vi "2D_Histogram_Selection.vi"() -> ()   [LabVIEW 2009]
uses:
  <vilib>/Utility/file.llb/Read From Spreadsheet File (DBL).vi
  <vilib>/Utility/file.llb/Write To Spreadsheet File (DBL).vi
panel:
  out "transposed array":dbl[][](array[numeric])
  out "array w/ subset deleted":dbl[](array[numeric])
  out "deleted portion":dbl[](array[numeric])
  in  "1-D Histogram?":bool
  out "1-D Histogram":cluster{dbl[], dbl[]}(graph)
  in  "Result File Dir":path=path "C:/Users/Habid/Documents/08_22_2013/08_22_2013/c6/25.7mV_3RR_2kHz_100mv_MC900/bcurve_selection_0.4"
  in  "Result File Name":string="beta_Histogram.txt"
  in  "Save 1-D":bool
  out "x+1":i32
  out "Cursor.Cursor Index 2":i32
  out "Cursor.Cursor Index":i32
  out "element":dbl
  out "Cursor.Cursor Position:Cursor X":dbl
  in  "Save":bool
  in  "Result File Name 2":string="1D_Histogram.txt"
  in  "Result File Dir 2":path
  out "Result":dbl[][](array[numeric])
  out "Row":i32
  out "Cursor 3":T1 {"Cursor.Cursor Z" format="%.2f"; "Cursor.Cursor Y" format="%.2f"; "Cursor.Cursor X" format="%.2f"}
  out "Cursor 2":T1 {"Cursor.Cursor Z" format="%.2f"; "Cursor.Cursor Y" format="%.2f"; "Cursor.Cursor X" format="%.2f"}
  out "Total 2D Histogram":dbl[][](graph)
  in  "Filename":path=path "C:/Users/Habid/Documents/08_22_2013/08_22_2013/c6/25.7mV_3RR_2kHz_100mv_MC900/bcurve_selection_0.4/2D_Histogram.txt"
  out "Cursor 0":T1 {"Cursor.Cursor Z" format="%.2f"; "Cursor.Cursor Y" format="%.2f"; "Cursor.Cursor X" format="%.2f"}
  out "Cursor 1":T1 {"Cursor.Cursor Z" format="%.2f"; "Cursor.Cursor Y" format="%.2f"; "Cursor.Cursor X" format="%.2f"}
  out "Intensity Graph":dbl[][](graph)
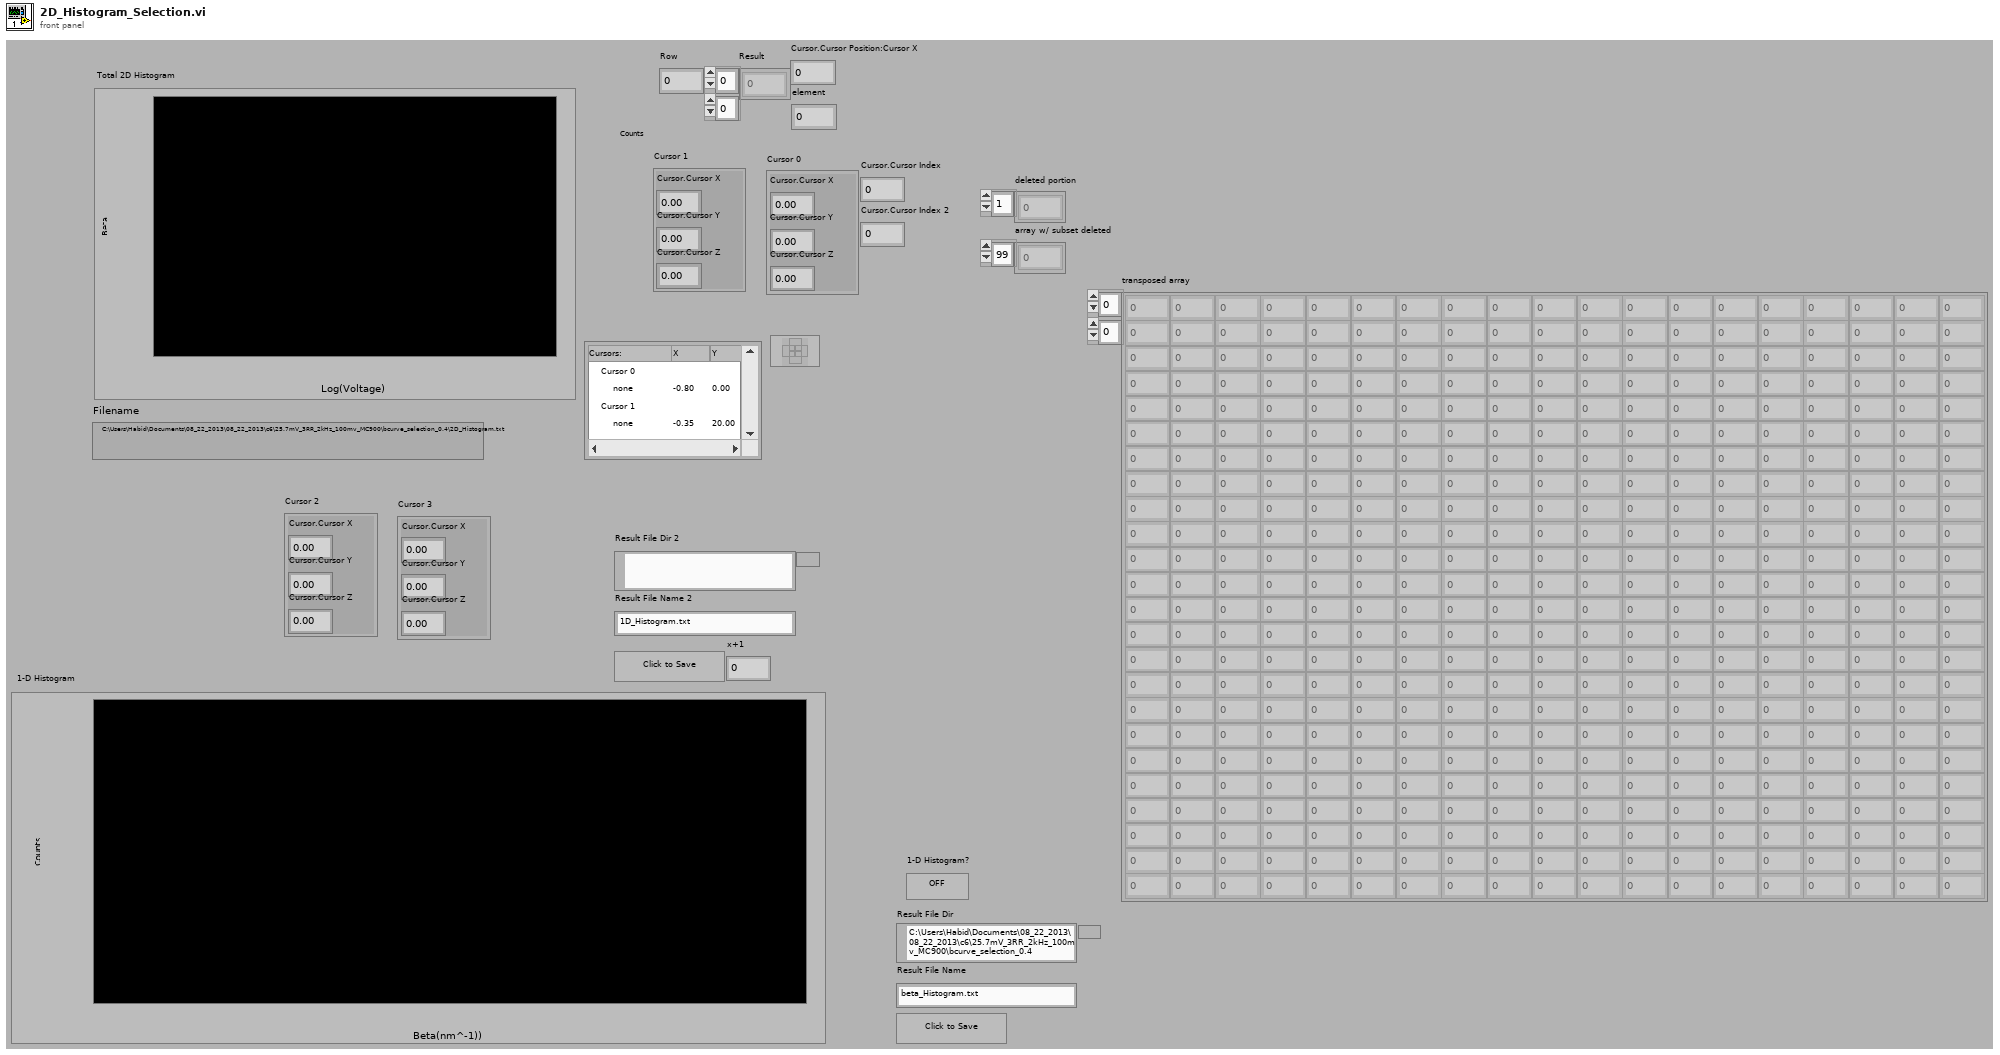
[diagram p1: front panel]
types:
  T1 = cluster{"Cursor.Cursor X":dbl, "Cursor.Cursor Y":dbl, "Cursor.Cursor Z":dbl}
  T2 = cluster{"Cursor.Cursor X":dbl, "Cursor.Cursor Y":dbl, dbl}
  T3 = cluster{"Cursor.Cursor X":dbl, "Cursor.Cursor Y":dbl, "number: 0 to 1":dbl}
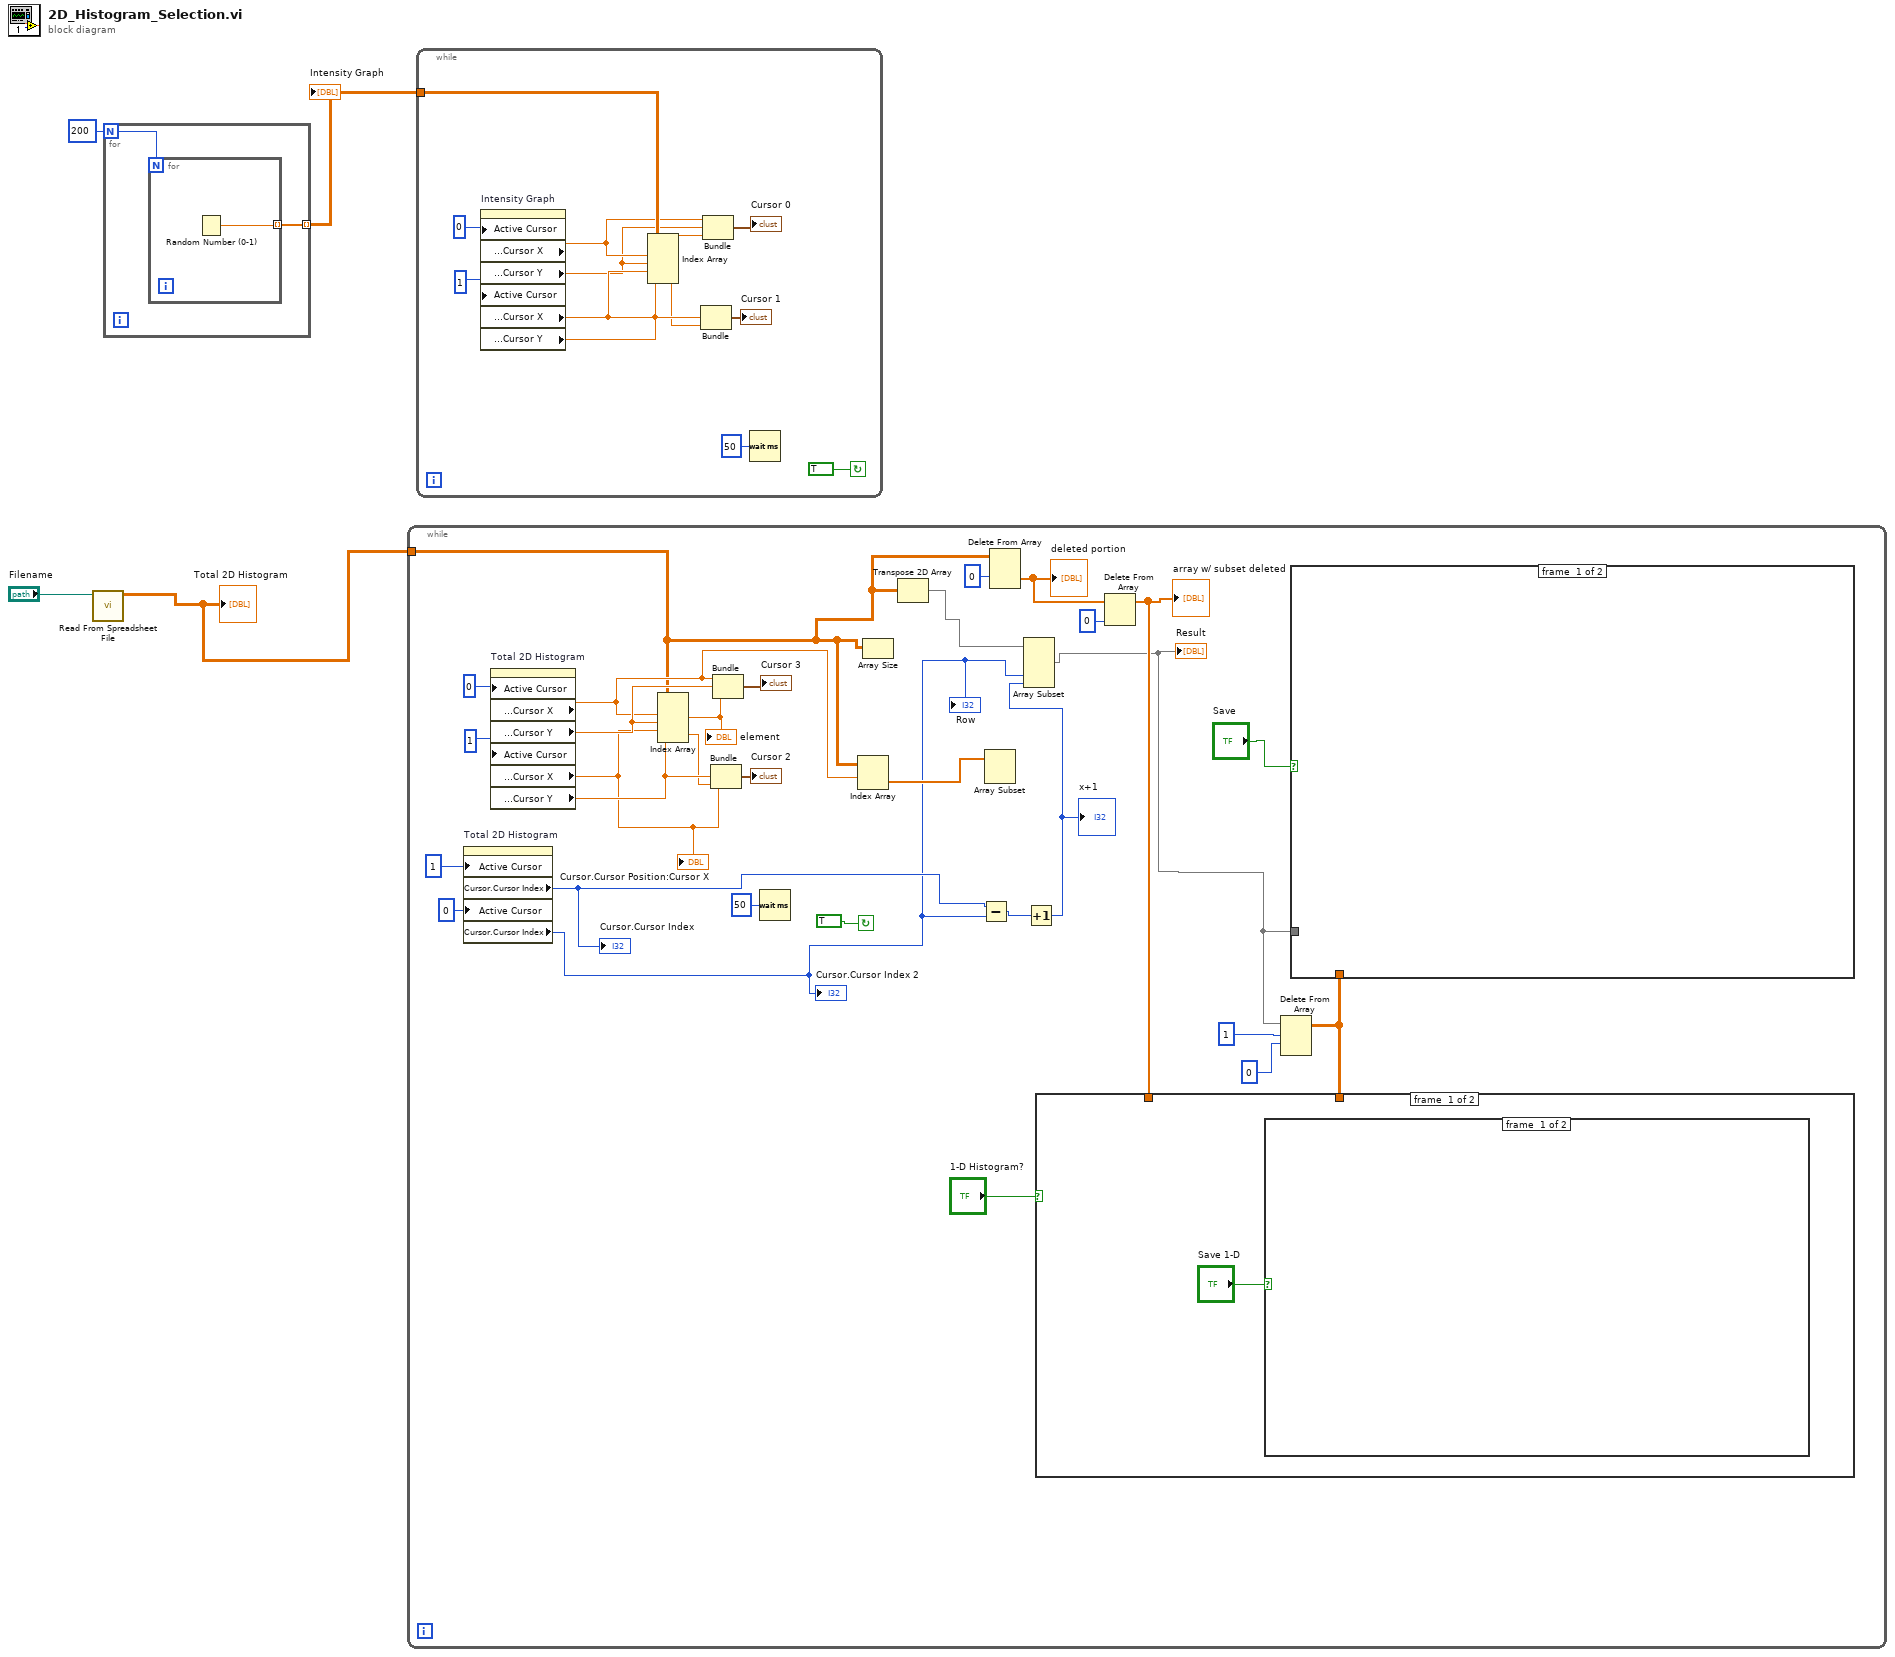
[diagram p0: block diagram]
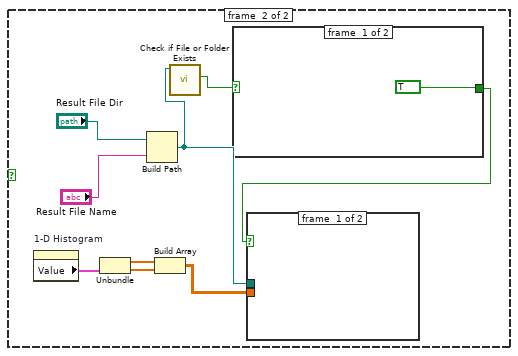
[diagram p2: hidden frame]
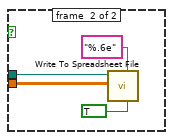
[diagram p3: hidden frame]
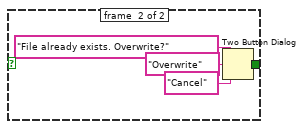
[diagram p4: hidden frame]
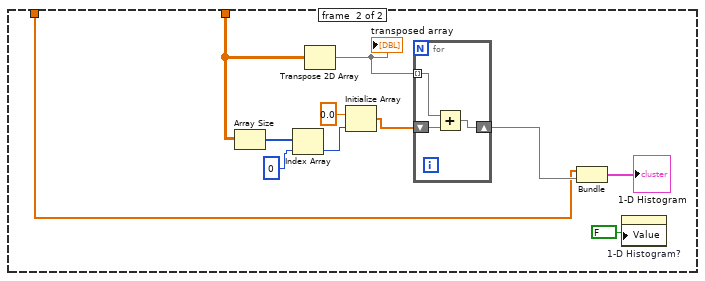
[diagram p5: hidden frame]
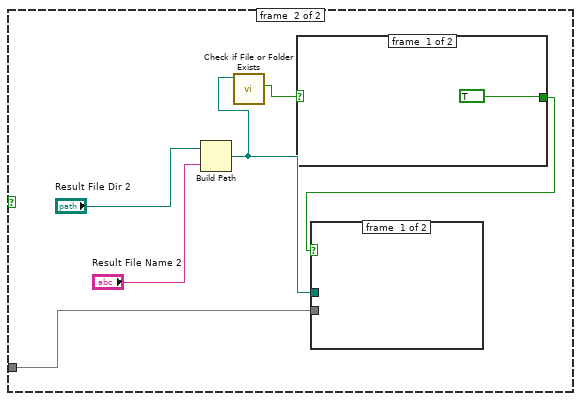
[diagram p6: hidden frame]
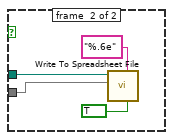
[diagram p7: hidden frame]
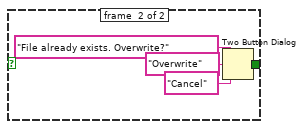
[diagram p8: hidden frame]
diagram:
  n1 = call-poly <vilib>:"Read From Spreadsheet File.vi"("file path (dialog if empty)"="Filename") -> ("all rows"=w1:dbl[][])  [unwired: 6 in, 4 out]
  "Total 2D Histogram" <- w1
  n2 = for {
    N: 200 -> [w6]
    tunnel: [w5] -> w3 mode=indexing
    n3 = for {
      N: w6 -> [_]
      tunnel: [w7] -> w5 mode=indexing
      n4 = Random Number (0-1)() -> (number: 0 to 1=w7:dbl)
    }
  }
  "Intensity Graph" <- w3
  n5 = while {
    tunnel: w1 -> [w13]
    stop <- TRUE continue-if-true
    n6 = property on="Total 2D Histogram" class="IntGraph (strict)"("Active Cursor"=u32 1, "Active Cursor"=u32 0) -> ("Cursor.Cursor Index"=w22:i32, "Cursor.Cursor Index"=w18:i32)  [unwired: 2 in, 2 out]
    "Row" <- w18
    "Cursor.Cursor Index" <- w22
    "Cursor.Cursor Index 2" <- w18
    n7 = property on="Total 2D Histogram" class="IntGraph (strict)"("Active Cursor"=u32 0, "Active Cursor"=u32 1) -> ("Cursor.Cursor Position:Cursor X"=w26:dbl, "Cursor.Cursor Position:Cursor Y"=w31:dbl, "Cursor.Cursor Position:Cursor X"=w27:dbl, "Cursor.Cursor Position:Cursor Y"=w35:dbl)  [unwired: 2 in, 2 out]
    "Cursor.Cursor Position:Cursor X" <- w27
    n8 = Index Array(array=w13, index (row) #1=w26, index (col) #1=w31, index (row) #2=w27, index (col) #2=w35) -> (element #1=w32:dbl, element #2=w34:dbl)
    "element" <- w32
    n9 = Bundle("Cursor.Cursor X"=w27, "Cursor.Cursor Y"=w35, w34) -> (→"Cursor 2":T2)  [unwired: 1 in]
    n10 = Bundle("Cursor.Cursor X"=w26, "Cursor.Cursor Y"=w31, w32) -> (→"Cursor 3":T2)  [unwired: 1 in]
    n11 = Wait (ms)(milliseconds to wait=u32 50) -> ()  [unwired: 1 out]
    n12 = Index Array(array=w13, index (row)=w26) -> (element=w28:dbl[])  [unwired: 1 in]
    n13 = Array Size(array=w13) -> ()  [unwired: 1 out]
    n14 = Transpose 2D Array(2D array=w13) -> (transposed array=w20:dbl[][])
    n15 = Subtract(x=w22, y=w18) -> (x-y=w21:i32)
    n16 = Array Subset(array=w28) -> ()  [unwired: 2 in, 1 out]
    n17 = Delete From Array(array=w13, index (row)=0) -> (deleted portion=w11:dbl[])  [unwired: 2 in, 1 out]
    "deleted portion" <- w11
    n18 = Increment(x=w21) -> (x+1=w19:i32)
    "x+1" <- w19
    n19 = Array Subset(array=w20, index (col)=w18, length (col)=w19) -> (w8:dbl[][])  [unwired: 2 in]
    "Result" <- w8
    n20 = Delete From Array(array=w11, index=0) -> (array with subset deleted=w9:dbl[])  [unwired: 1 in, 1 out]
    "array w/ subset deleted" <- w9
    n21 = Delete From Array(array=w8, length=1, index (row)=0 ("disabled index (col)")) -> (array with subset deleted=w14:dbl[][])  [unwired: 1 in, 1 out]
    n22 = case shown="True" "1-D Histogram?" {
      tunnel: w14 -> [_ w64]
      tunnel: w9 -> [_ w59]
      frame #0 {
        n23 = case shown="True" "Save 1-D" {
          frame #0 {
          }
          frame #1 {
            n24 = property on="1-D Histogram" class="XYGraph (strict)"() -> ("Value"=w48:cluster{dbl[], dbl[]})  [unwired: 2 in, 2 out]
            n25 = Unbundle(w48) -> (w47:dbl[], w46:dbl[])
            n26 = Build Path(base path="Result File Dir", name or relative path="Result File Name") -> (appended path=w41:path)
            n27 = Build Array(w47, w46) -> (w40:dbl[][])
            n28 = call <vilib>:"Check if File or Folder Exists.vi"("path"=w41) -> ("file or folder exists?"=w43:bool)  [unwired: 8 in, 2 out]
            n29 = case shown="True" w43 {
              tunnel: [TRUE ("T button?") w54] -> w42
              frame #0 {
              }
              frame #1 {
                n30 = Two Button Dialog(message="File already exists. Overwrite?", 1:"Cancel" ("F button name (\"Cancel\")"), 2:"Overwrite" ("T button name (\"OK\")")) -> (T button?=w54:bool)
              }
            }
            n31 = case shown="True" w42 {
              tunnel: w40 -> [_ w50]
              tunnel: w41 -> [_ w51]
              frame #0 {
              }
              frame #1 {
                n32 = call-poly <vilib>:"Write To Spreadsheet File.vi"("transpose? (no:F)"=TRUE, "format (%.3f)"="%.6e", "2D data"=w50, "file path (dialog if empty)"=w51) -> ()  [unwired: 4 in, 1 out]
              }
            }
          }
        }
      }
      frame #1 {
        n33 = Array Size(array=w64) -> (size(s)=w63:i32[])
        n34 = Index Array(array=w63, index=0) -> (element=w62:i32)
        n35 = Transpose 2D Array(2D array=w64) -> (transposed array=w65:dbl[][])
        "transposed array" <- w65
        n36 = Initialize Array(0.0 ("element"), w62) -> (w60:dbl[])
        n37 = for {
          tunnel: w65 -> [w71] mode=indexing
          shift-right: [w69] -> w68
          shift-left: w60 -> [w70]
          n38 = Add(x=w71, y=w70) -> (x+y=w69:dbl[])
        }
        n39 = Bundle("all rows"=w59, w68) -> (→"1-D Histogram":cluster{"all rows":dbl[], dbl[]})  [unwired: 1 in]
        n40 = property on="1-D Histogram?" class="Bool (strict)"("Value"=FALSE ("1-D Histogram?")) -> ()  [unwired: 2 in, 2 out]
      }
    }
    n41 = case shown="True" "Save" {
      tunnel: w14 -> [_ _]
      tunnel: w8 -> [_ w72]
      frame #0 {
      }
      frame #1 {
        n42 = Build Path(base path="Result File Dir 2", name or relative path="Result File Name 2") -> (appended path=w75:path)
        n43 = call <vilib>:"Check if File or Folder Exists.vi"("path"=w75) -> ("file or folder exists?"=w77:bool)  [unwired: 8 in, 2 out]
        n44 = case shown="True" w77 {
          tunnel: [TRUE ("T button?") w83] -> w76
          frame #0 {
          }
          frame #1 {
            n45 = Two Button Dialog(message="File already exists. Overwrite?", 1:"Cancel" ("F button name (\"Cancel\")"), 2:"Overwrite" ("T button name (\"OK\")")) -> (T button?=w83:bool)
          }
        }
        n46 = case shown="True" w76 {
          tunnel: w75 -> [_ w80]
          tunnel: w72 -> [_ w78]
          frame #0 {
          }
          frame #1 {
            n47 = call-poly <vilib>:"Write To Spreadsheet File.vi"("transpose? (no:F)"=TRUE, "format (%.3f)"="%.6e", "2D data"=w78, "file path (dialog if empty)"=w80) -> ()  [unwired: 4 in, 1 out]
          }
        }
      }
    }
  }
  n48 = while {
    tunnel: w3 -> [w95]
    stop <- TRUE continue-if-true
    n49 = property on="Intensity Graph" class="IntensityGraph (strict)"("Active Cursor"=u32 0, "Active Cursor"=u32 1) -> ("Cursor.Cursor Position:Cursor X"=w89:dbl, "Cursor.Cursor Position:Cursor Y"=w88:dbl, "Cursor.Cursor Position:Cursor X"=w94:dbl, "Cursor.Cursor Position:Cursor Y"=w93:dbl)  [unwired: 2 in, 2 out]
    n50 = Index Array(array=w95, index (row) #1=w89, index (col) #1=w88, index (row) #2=w94, index (col) #2=w93) -> (element #1=w90:dbl, element #2=w92:dbl)
    n51 = Bundle("Cursor.Cursor X"=w94, "Cursor.Cursor Y"=w93, "number: 0 to 1"=w92) -> (→"Cursor 1":T3)  [unwired: 1 in]
    n52 = Bundle("Cursor.Cursor X"=w89, "Cursor.Cursor Y"=w88, "number: 0 to 1"=w90) -> (→"Cursor 0":T3)  [unwired: 1 in]
    n53 = Wait (ms)(milliseconds to wait=u32 50) -> ()  [unwired: 1 out]
  }
